vi "display permission to classification.vi"(11 "display permissions":T1) -> (3 "channel classification":T2)   [LabVIEW 2014]
uses:
  <vilib>/NI/Tag Bus Module Framework/channel/channel classification.ctl
  permissions.ctl
  <vilib>/NI/Tag Bus Module Framework/channel/TBM channel.lvclass
  Tagbus PID Module editor node.lvclass
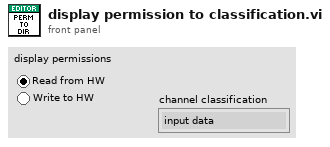
[diagram p1: front panel]
types:
  T1 = typedef "Tagbus PID Module editor node.lvclass/permissions.ctl" = enum32{"Read from HW", "Write to HW"}
  T2 = typedef "TBM channel.lvclass/channel classification.ctl" = enum16{"input data", "output data", "processing parameter", "processing result"}
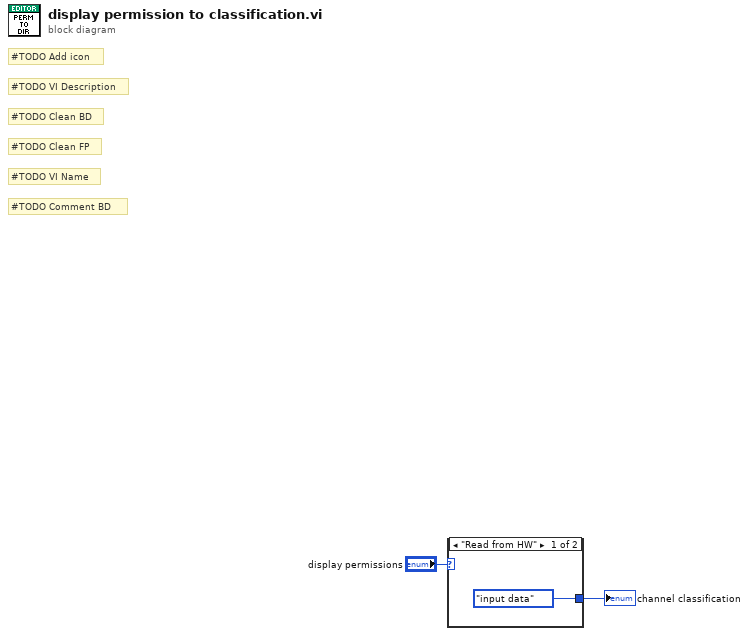
[diagram p0: block diagram]
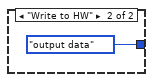
[diagram p2: hidden frame]
diagram:
  # "#TODO Comment BD"
  # "#TODO VI Name"
  # "#TODO Clean FP"
  # "#TODO Clean BD"
  # "#TODO VI Description"
  # "#TODO Add icon"
  n1 = case shown="\"Read from HW\"" "display permissions" {
    tunnel: [channel_classification."input data" ("channel classification") channel_classification."output data" ("channel classification")] -> w2
    frame "Read from HW" {
    }
    frame "Write to HW" {
    }
  }
  "channel classification" <- w2
